vi "Check Package.vi"(8 "error in (no error)":errorcluster, 10 "Package":refnum<class "PackageAbstract.lvclass">, 11 "UpdateAction in":refnum<class "DependAction.lvclass">) -> (0 "error out":errorcluster, 2 "Problems":string[](array[string]), 3 "UpdateAction out":refnum<class "DependAction.lvclass">)   [LabVIEW 2020, in "GPackTools.lvlib" / "DependAction.lvclass"]
uses:
  DependAction.lvclass
  GPack/PackageAbstract/PackageAbstract.lvclass
  C:/dev/lv20CE/lv-gpack/GPack/Package/Package.lvclass
  GPack/Package/Package.lvclass
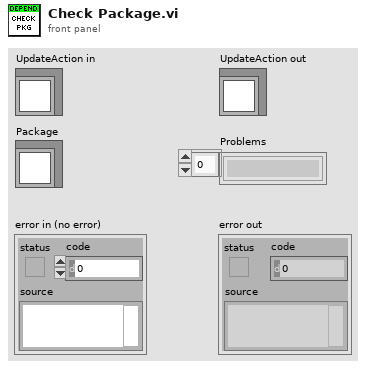
[diagram p1: front panel]
types:
  T1 = typedef "GPack.lvlib/Package Info.ctl" = cluster{"Name":string, "Type":string, "Host":string, "Path":string, "Branch":string, "Version":string, "License":string}
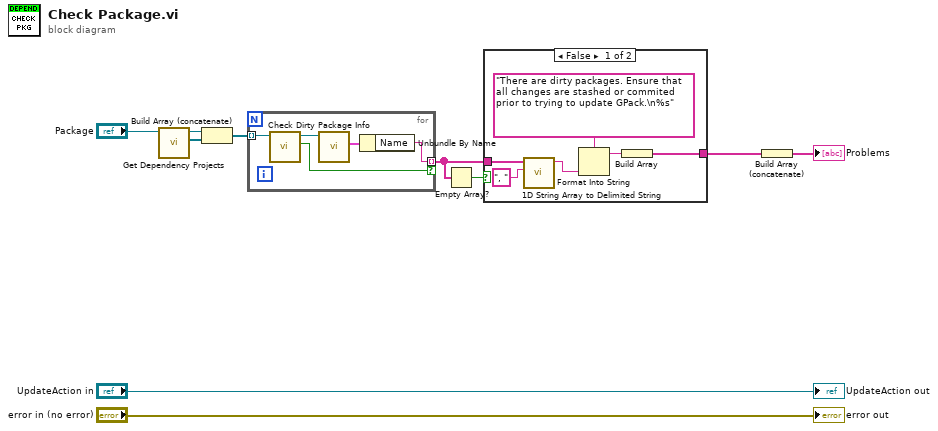
[diagram p0: block diagram]
diagram:
  n1 = call "Get Dependency Projects.vi"("PackageAbstract in"="Package") -> ("Dependencies"=w7:refnum<class "Package.lvclass">[], "PackageAbstract out"=w8:refnum<class "PackageAbstract.lvclass">)  [unwired: 8 in, 1 out]
  n2 = Build Array (concatenate)(w8, w7) -> (w6:refnum<class "Package.lvclass">[])
  n3 = for {
    tunnel: w6 -> [w15] mode=indexing
    tunnel: [w12] -> w4 mode=indexing if=w11
    n4 = call-dynamic "Check Dirty.vi"("Package in"=w15) -> ("Dirty"=w11:bool, "Package out"=w14:refnum<class "Package.lvclass">)  [unwired: 8 in, 1 out]
    n5 = call-dynamic "Package Info.vi"("Package in"=w14) -> ("Package Info"=w13:T1)  [unwired: 8 in, 2 out]
    n6 = Unbundle By Name(w13) -> ("Name"=w12:string)
  }
  n7 = Empty Array?(array=w4) -> (empty?=w5:bool)
  n8 = case shown="False" w5 {
    tunnel: w4 -> [w21 _]
    tunnel: [w16 _] -> w3
    frame False {
      n9 = call <vilib>:"1D String Array to Delimited String.vi"("delimiter"=", ", "string array"=w21) -> ("delimited string"=w19:string)  [unwired: 9 in]
      n10 = Format Into String(format string="There are dirty packages. Ensure that all changes are stashed or commited prior to trying to update GPack.\n%s", w19) -> (resulting string=w17:string)  [unwired: 2 in, 1 out]
      n11 = Build Array(w17) -> (w16:string[])
    }
    frame True {
    }
  }
  n12 = Build Array (concatenate)(w3) -> (→"Problems":string[])
  "error out" <- "error in (no error)"
  "UpdateAction out" <- "UpdateAction in"
